vi "FTW-Messenger-Construct.vi"(0 "Messenger Type":refnum<class "FTW-Messenger.lvclass">, 11 "error in":errorcluster) -> (4 "Messenger":refnum<class "FTW-Messenger.lvclass">, 15 "error out":errorcluster)   [LabVIEW 2014, in "FTW-Messenger.lvclass"]
uses:
  FTW-Messenger.lvclass
  Message/FTW-Message.lvclass
panel:
  # "Inputs"
  # "Outputs"
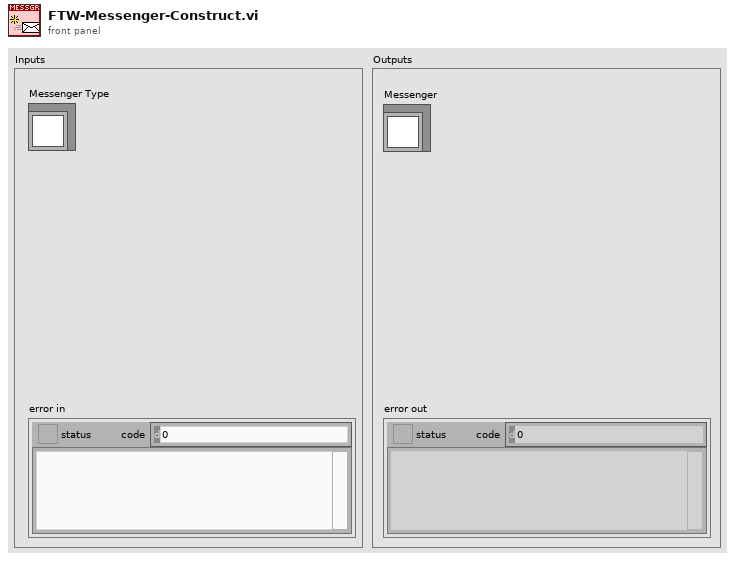
[diagram p1: front panel]
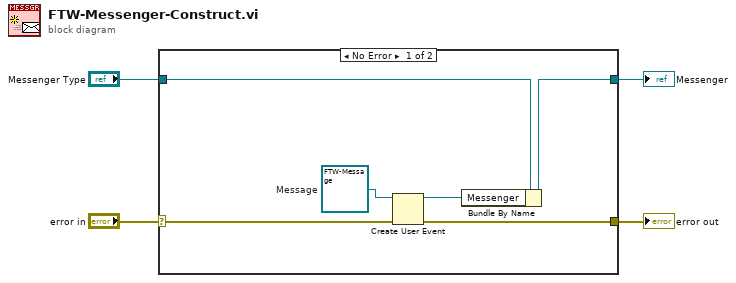
[diagram p0: block diagram]
diagram:
  n1 = case shown="No Error" "error in" {
    selector: "error in" -> [w10 w12]
    tunnel: [w7 w12] -> w2
    tunnel: [w8 w11] -> w3
    tunnel: "Messenger Type" -> [w9 w11]
    frame No Error {
      w6 = refnum<class "FTW-Message.lvclass"> refnum  # Message
      n2 = Create User Event(user event datatype=w6, error in=w10) -> (user event=w5:refnum<user-event>, error out=w7:errorcluster)
      n3 = Bundle By Name(cluster=w9, "Messenger"=w5) -> (w8:refnum<class "FTW-Messenger.lvclass">)
    }
    frame Error {
    }
  }
  "Messenger" <- w3
  "error out" <- w2
